vi "Set Button Color.vi"(8 "error in (no error)":errorcluster, 10 "Color Theme":T1={"Primary"=6323595, "Primary Light"=13621468, "Primary Dark"=4545124, "Accent"=10395294, "Primary Text"=2171169, "Secondary Text"=7697781}, 11 "Reference in":refnum<vi>) -> (0 "error out":errorcluster, 3 "Reference out":refnum<vi>)   [LabVIEW 2020, in "Execution UI V2.lvclass"]
uses:
  Execution UI V2.lvclass
  TypeDefs/Color Theme.ctl
  Execution UI V2.lvclass/Execution UI V2.ctl
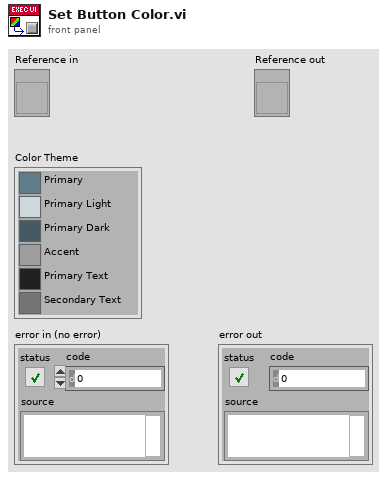
[diagram p1: front panel]
types:
  T1 = typedef "Execution UI V2.lvclass/Color Theme.ctl" = cluster{"Primary":u32, "Primary Light":u32, "Primary Dark":u32, "Accent":u32, "Primary Text":u32, "Secondary Text":u32}
  T2 = cluster{"Primary Light":u32, "Primary Light":u32}
  T3 = cluster{"Primary Dark":u32, "Primary Dark":u32}[]
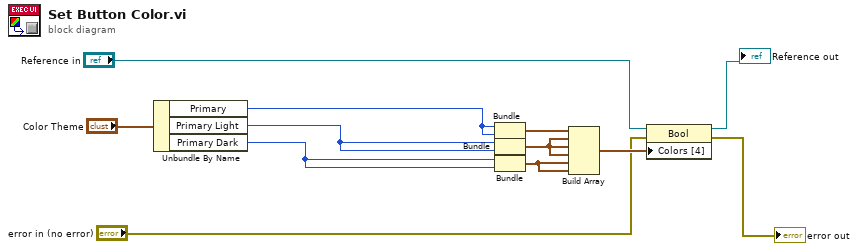
[diagram p0: block diagram]
diagram:
  n1 = Unbundle By Name("Color Theme") -> ("Primary"=w11:u32, "Primary Light"=w9:u32, "Primary Dark"=w10:u32)
  n2 = Bundle("Primary"=w11, "Primary"=w11) -> (w8:cluster{"Primary":u32, "Primary":u32})  [unwired: 1 in]
  n3 = Bundle("Primary Light"=w9, "Primary Light"=w9) -> (w7:T2)  [unwired: 1 in]
  n4 = Bundle("Primary Dark"=w10, "Primary Dark"=w10) -> (w6:cluster{"Primary Dark":u32, "Primary Dark":u32})  [unwired: 1 in]
  n5 = Build Array(w8, w7, w7, w7, w6, w6) -> (w5:T3)
  n6 = property on="Property Node" class="Bool"(reference="Reference in", error in="error in (no error)", "Colors [4]"=w5) -> (reference out=→"Reference out":refnum<vi>, error out=→"error out":errorcluster)
